vi "DAC Save Results.vi"(8 "error in":errorcluster, 9 "Log Details?":bool, 10 "tdms file":refnum<k34>, 11 "DAC Inverter in":refnum<class "DAC Inverter.lvclass">) -> (0 "error out":errorcluster)   [LabVIEW 2019, in "DAC.lvlib" / "DAC Inverter.lvclass"]
uses:
  DAC Inverter.lvclass
  C:/Users/krio/Documents/LV_Projects/test-stand/App/DAC/DAC.lvclass
  DAC.lvclass/DAC.ctl
  DAC Inverter.lvclass/DAC Inverter.ctl
  DAC.lvclass
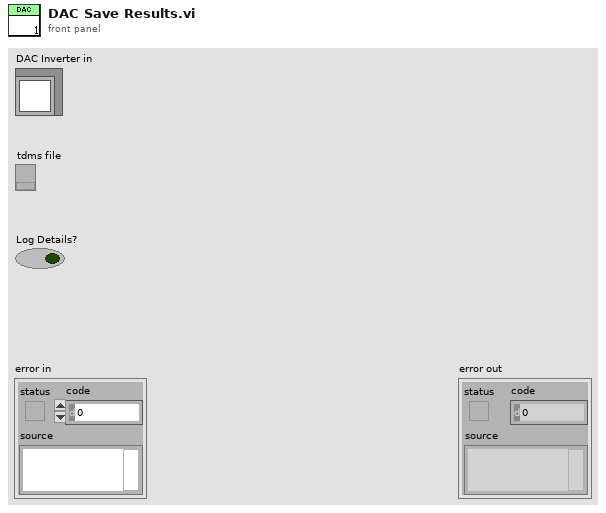
[diagram p1: front panel]
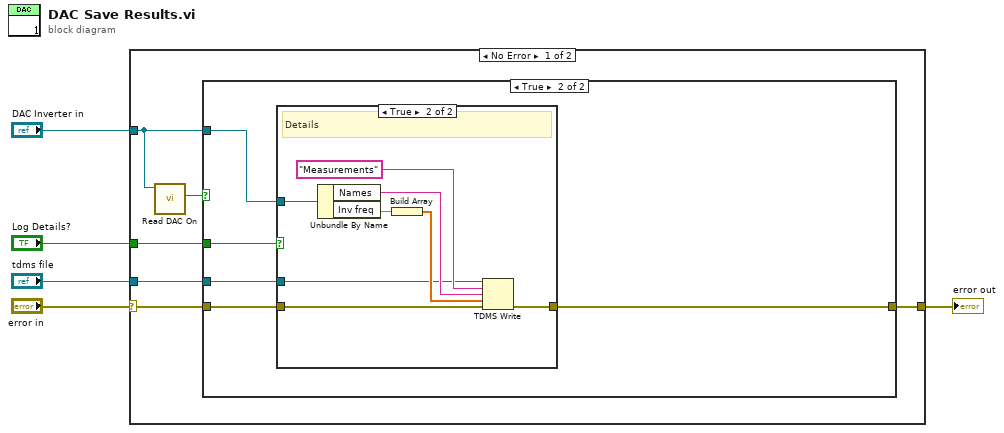
[diagram p0: block diagram]
diagram:
  n1 = case shown="No Error" "error in" {
    selector: "error in" -> [w8 w27]
    tunnel: "DAC Inverter in" -> [w11 _]
    tunnel: "tdms file" -> [w9 _]
    tunnel: [w7 w27] -> w2
    tunnel: "Log Details?" -> [w6 _]
    frame No Error {
      n2 = call "Read DAC On.vi"("DAC in"=w11) -> ("DAC On"=w10:bool)  [unwired: 8 in, 2 out]
      n3 = case shown="True" w10 {
        tunnel: w11 -> [_ w17]
        tunnel: w9 -> [_ w16]
        tunnel: w8 -> [w12 w14]
        tunnel: [w12 w15] -> w7
        tunnel: w6 -> [_ w13]
        frame False {
        }
        frame True {
          n4 = case shown="True" w13 {
            tunnel: w17 -> [_ w26]
            tunnel: w16 -> [_ w19]
            tunnel: [w18 w25] -> w15
            tunnel: w14 -> [w18 w20]
            frame False {
            }
            frame True {
              # "Details"
              n5 = Unbundle By Name(w26) -> ("Names"=w21:string, "Inv freq"=w23:dbl)
              n6 = Build Array(w23) -> (w22:dbl[])
              n7 = TDMS Write(0:w19, 5:"Measurements" ("group name in (Untitled)"), 7:w21, 9:w22, 11:w20) -> (15:w25:errorcluster)  [unwired: 1 in, 3 out]
            }
          }
        }
      }
    }
    frame Error {
    }
  }
  "error out" <- w2
